vi "Create (OpenVINO).vi"(5 "Backends (Default: DEFAULT)":T5, 6 "Image Handling Properties":T1, 7 "Target (Default: CPU)":T4, 8 "error in (no error)":errorcluster, 10 "Config (*.xml)":path, 11 "OpenVINO Model (*.bin or *.onnx)":path) -> (0 "error out":errorcluster, 3 "DNN Detection Model":refnum<class "DNN Detection Model.lvclass">)   [LabVIEW 2020, in "feature_detection.lvlib" / "DNN Detection Model.lvclass"]
uses:
  DNN Detection Model.lvclass
  Backends.ctl
  Targets.ctl
  Model Parameters.ctl
  common/Image Size (Integer).ctl
  common/Object Point (Float).ctl
  DNN Detection Model.lvclass/DNN Detection Model.ctl
  Path to String.vi
  <vilib>/Utility/error.llb/Error Cluster From Error Code.vi
  common/common.lvlib
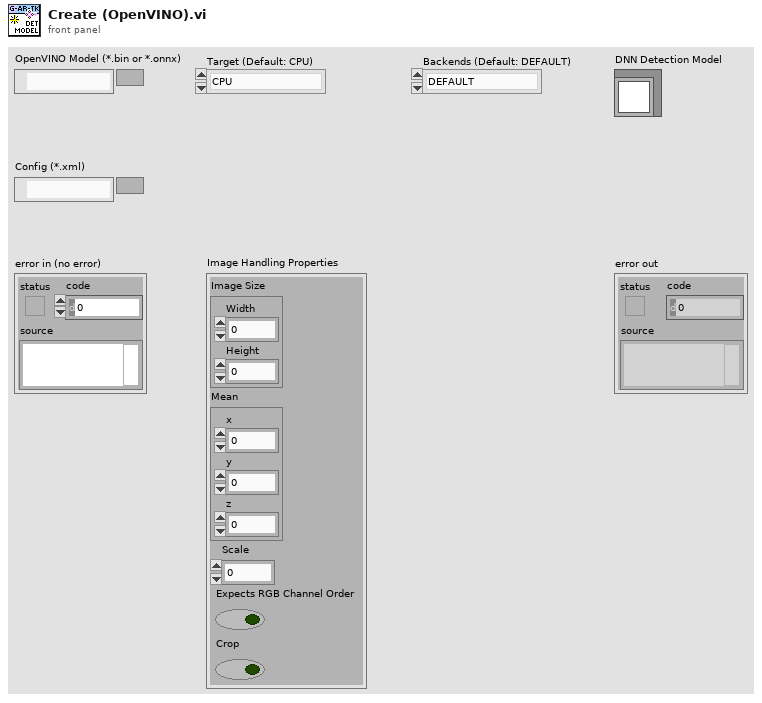
[diagram p1: front panel]
types:
  T1 = typedef "feature_detection.lvlib/DNN Detection Model.lvclass/Model Parameters.ctl" = cluster{"Image Size":T2, "Mean":T3, "Scale":dbl, "Expects RGB Channel Order":bool, "Crop":bool}
  T2 = typedef "common.lvlib/Image Size (Integer).ctl" = cluster{"Width":u16, "Height":u16}
  T3 = typedef "common.lvlib/Object Point (Float).ctl" = cluster{"x":dbl, "y":dbl, "z":dbl}
  T4 = typedef "feature_detection.lvlib/DNN Detection Model.lvclass/Targets.ctl" = enum16{"CPU", "OPENCL", "OPENCL_FP16", "MYRIAD", "VULKAN", "FPGA", "CUDA", "CUDA_FP16", "HDDL", "NPU", "CPU_FP16"}
  T5 = typedef "feature_detection.lvlib/DNN Detection Model.lvclass/Backends.ctl" = enum8{"DEFAULT", "HALIDE", "INFERENCE_ENGINE", "OPENCV", "VKCOM", "CUDA", "WEBNN", "TIMVX", "CANN"}
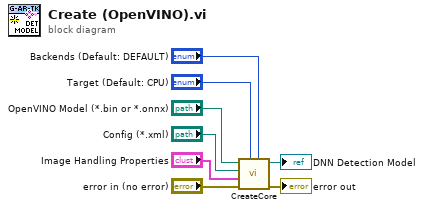
[diagram p0: block diagram]
diagram:
  n1 = call "CreateCore.vi"("Backends"="Backends (Default: DEFAULT)", "Target"="Target (Default: CPU)", "error in (no error)"="error in (no error)", "Model Properties"="Image Handling Properties", "Config File"="Config (*.xml)", "Model File"="OpenVINO Model (*.bin or *.onnx)") -> ("error out"=→"error out":errorcluster, "DNN Detection Model"=→"DNN Detection Model":refnum<class "DNN Detection Model.lvclass">)  [unwired: 4 in]
